vi "OpenDependencyListExportVIs.vi"   [LabVIEW 2020]
types:
  T1 = enum32{"Invalid", "Standard", "Closed", "Hidden", "Minimized", "Maximized"}
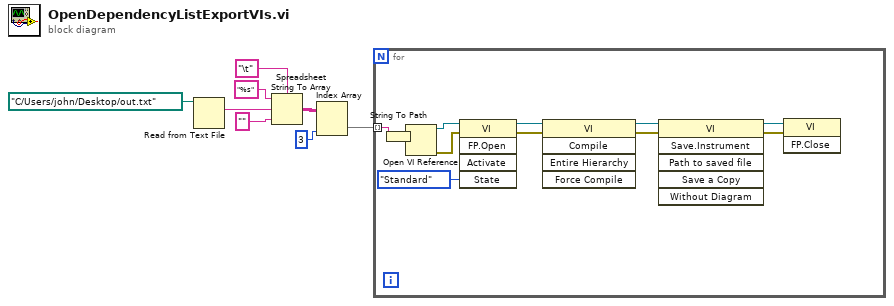
[diagram p0: block diagram]
diagram:
  n1 = Read from Text File(file (use dialog)=path "C:/Users/john/Desktop/out.txt") -> (text=w5:string)  [unwired: 3 in, 3 out]
  n2 = Spreadsheet String To Array(delimiter (Tab)="\t" ("delimiter"), format string="%s", spreadsheet string=w5, array type (2D Dbl)="") -> (array=w6:string[][])
  n3 = Index Array(array=w6, index (col)=3 ("index")) -> (element=w1:string[])  [unwired: 1 in]
  n4 = for {
    tunnel: w1 -> [w19] mode=indexing
    n5 = String To Path(string=w19) -> (path=w18:path)
    n6 = Open VI Reference(vi path=w18) -> (vi reference=w17:refnum<vi>, error out=w15:errorcluster)  [unwired: 5 in]
    n7 = invoke class="VI" method="FP.Open"(reference=w17, error in=w15, "State"=T1."Standard") -> (reference out=w14:refnum<vi>, error out=w13:errorcluster)  [unwired: 2 in, 3 out]
    n8 = invoke class="VI" method="Compile"(reference=w14, error in=w13) -> (reference out=w12:refnum<vi>, error out=w11:errorcluster)  [unwired: 3 in, 3 out]
    n9 = invoke class="VI" method="Save.Instrument"(reference=w12, error in=w11) -> (reference out=w10:refnum<vi>, error out=w9:errorcluster)  [unwired: 4 in, 4 out]
    n10 = invoke class="VI" method="FP.Close"(reference=w10, error in=w9) -> ()  [unwired: 1 in, 3 out]
  }
